vi "Transceiver PPL Test.vi"() -> ()   [LabVIEW 2017]
uses:
  Built/DSF.Engine.lvlibp/Engine/Classes/Transceiver/DSF.Engine.Transceiver Loader.lvclass
  Built/DSF.Engine.lvlibp/Engine/Classes/Transceiver/DSF.Engine.Transceiver.lvclass
panel:
  out "Array":string[](array[string])
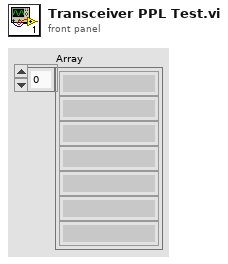
[diagram p1: front panel]
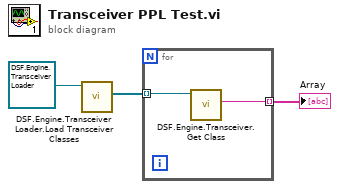
[diagram p0: block diagram]
diagram:
  n1 = call "DSF.Engine.Transceiver Loader.Load Transceiver Classes.vi"("Transceiver Loader in"=refnum<class "DSF.Engine.Transceiver Loader.lvclass"> refnum) -> ("Transceivers"=w3:refnum<class "DSF.Engine.Transceiver.lvclass">[])  [unwired: 8 in, 2 out]
  n2 = for {
    tunnel: w3 -> [w5] mode=indexing
    tunnel: [w4] -> w2 mode=indexing
    n3 = call-dynamic "DSF.Engine.Transceiver.Get Class.vi"("Transceiver in"=w5) -> ("class"=w4:string)  [unwired: 8 in, 2 out]
  }
  "Array" <- w2
